vi "steup-CS-scan-fpga.vi"() -> ()   [LabVIEW 2017]
uses:
  fpga_VIs/controls/supervisor-params.ctl
  controls/z-axis-params_v4_prescan.ctl
  controls/TF-params.ctl
  fpga_VIs/fpga_subVIs_ssxy/fixed-point-ss/typeDefs/FXPControlParams-ss-xy.ctl
  fpga_interface_lib/fpga_interface_types/cs-scan-inputs-TYPE.ctl
  <vilib>/rvi/interface/common/niFpgaWaitOnOcc.vi
  <vilib>/Utility/error.llb/Error Cluster From Error Code.vi
  <vilib>/rvi/errors/niLvFpgaAdjustHostInterfaceError.vi
  <vilib>/rvi/interface/nirviMethod/nirviMethod.xnode
  <vilib>/rvi/interface/nirviReadWriteControl/nirviReadWriteControl.xnode
  fpga_interface_lib/fpga_interface.lvlib
  <vilib>/FPGAPlugInAG/Dynamic/niLvFpga_ConfigureFifo_Dynamic.vi
  <vilib>/rvi/errors/niLvFpgaMergeErrorWithErrorCode.vi
  NiFpgaLv.dll
  <vilib>/rvi/interface/Simulation/niFpgaSimulationCallBeginRW.vi
  <vilib>/FPGAPlugInAG/Dynamic/niLvFpga_WriteFifo_Dynamic.vi
panel:
  out "Empty Elements Remaining":u32
  out "error out":errorcluster
  out "FPGA Interface":T1
  in  "Control-matrices":sgl[](array[numeric])
  out "Actual Depth 3":u32
  out "Actual Depth 2":u32
  out "Actual Depth":u32
  in  "error in":errorcluster
  in  "ControlParamsLin-ss":T2={"umax"=3.0, "Ns_obs/cntrl"=0, "ref_f_VEC"=[0.0, 0.0], "du_max"=0.0, "Nbar"=0.0, "Nhyst"=0, "Nsat"=0, "Ndrift+1"=0, "Ki-y"=0.01}
  in  "z_axis_params":T3={"z_u_max"=5.0, "setpoint-scan"=-0.3000030517578125, "Ki-scan"=0.02, "uz_safe"=0.0, "Kiz_down"=0.02, "setpoint-up"=-0.899993896484375, "TF-params"={"TF-order"=0, "Num"=[0.0, 0.0, 0.0, 0.0, 0.0, 0.0, 0.0, 0.0, 0.0], "Den"=[0.0, 0.0, 0.0, 0.0, 0.0, 0.0, 0.0, 0.0, 0.0]}, "do-Dz"=FALSE, "PID-while-xy-move"=FALSE} {"Kiz_down" format="%#_13g"; "Ki-scan" min=0 max=0.4 step=0.0025; "z_u_max" format="%#_13g"}
  in  "state-machine-params":T5={"xy settled-samples\n threshold"=15, "xy error-threshold"=0.01, "zup-err-threshold"=0.10000228881835938, "prescan-samples"=5000, "TOL"=0.3, "collect all"=TRUE, "numEntities"=0} {"TOL" format="%#_13g"}
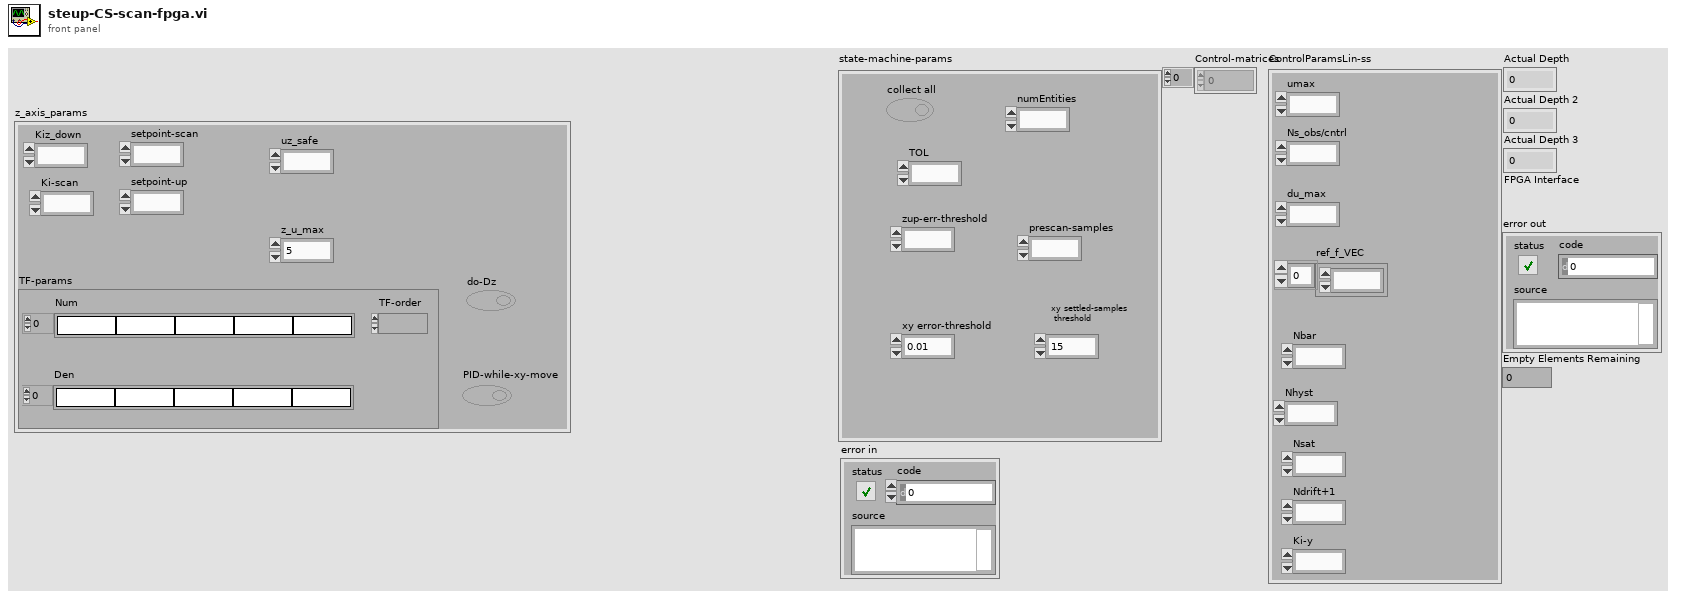
[diagram p1: front panel]
types:
  T1 = typedef "fpga_interface.lvlib/cs-scan-inputs-TYPE.ctl" = refnum<k20>
  T2 = typedef "FXPControlParams-ss-xy.ctl" = cluster{"umax":fxp<+/-,18,5>, "Ns_obs/cntrl":u8, "ref_f_VEC":fxp<+/-,32,5>[], "du_max":fxp<+/-,18,5>, "Nbar":fxp<+/-,32,5>, "Nhyst":u8, "Nsat":u8, "Ndrift+1":u8, "Ki-y":sgl}
  T3 = typedef "z-axis-params_v4_prescan.ctl" = cluster{"z_u_max":sgl, "setpoint-scan":fxp<+/-,32,16>, "Ki-scan":sgl, "uz_safe":fxp<+/-,16,5>, "Kiz_down":sgl, "setpoint-up":fxp<+/-,32,16>, "TF-params":T4, "do-Dz":bool, "PID-while-xy-move":bool}
  T4 = typedef "TF-params.ctl" = cluster{"TF-order":i16, "Num":sgl[], "Den":sgl[]}
  T5 = typedef "supervisor-params.ctl" = cluster{"xy settled-samples\n threshold":i16, "xy error-threshold":sgl, "zup-err-threshold":fxp<+,24,5>, "prescan-samples":i16, "TOL":sgl, "collect all":bool, "numEntities":i16}
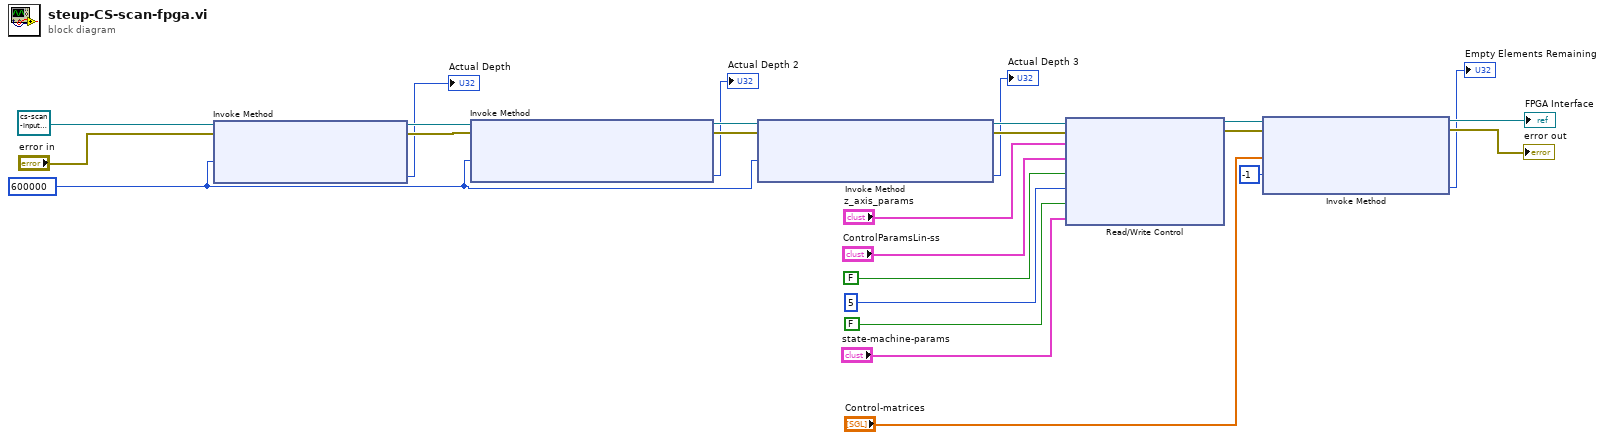
[diagram p0: block diagram]
diagram:
  w15 = 600000
  n1 = xnode "Invoke Method"("FPGA VI Reference In"=T1 refnum ("FPGA Interface"), "error in"="error in", "Requested Depth"=w15) -> ("FPGA VI Reference Out"=w19:T1, "error out"=w18:errorcluster, "Actual Depth"=→"Actual Depth":u32)
  n2 = xnode "Invoke Method"("FPGA VI Reference In"=w19, "error in"=w18, "Requested Depth"=w15) -> ("FPGA VI Reference Out"=w25:T1, "error out"=w24:errorcluster, "Actual Depth"=→"Actual Depth 2":u32)
  n3 = xnode "Invoke Method"("FPGA VI Reference In"=w25, "error in"=w24, "Requested Depth"=w15) -> ("FPGA VI Reference Out"=w23:T1, "error out"=w22:errorcluster, "Actual Depth"=→"Actual Depth 3":u32)
  n4 = xnode "Read/Write Control"("FPGA VI Reference In"=w23, "error in"=w22, "z_axis_params"="z_axis_params", "ControlParams-ss-xy"="ControlParamsLin-ss", "trigger-0"=FALSE, "num-log-channels"=u32 5 ("y"), "ABORT"=FALSE, "state-machine-params"="state-machine-params") -> ("FPGA VI Reference Out"=w21:T1, "error out"=w20:errorcluster)
  n5 = xnode "Invoke Method"("FPGA VI Reference In"=w21, "error in"=w20, "Data"="Control-matrices", "Timeout (ms)"=-1) -> ("FPGA VI Reference Out"=→"FPGA Interface":T1, "error out"=→"error out":errorcluster, "Empty Elements Remaining"=→"Empty Elements Remaining":u32)
